vi "Mode Scan Engine.vi"() -> ()   [LabVIEW 2016]
uses:
  <vilib>/vision/Image Controls.llb/IMAQ Image.ctl
  Hardware Configuration/Hardware Configuration Controls/Standard Action.ctl
  Device Library/Cameras/Hamamatsu/Orca Flash/Orca Flash Controls/Orca Flash Actions.ctl
  Hardware Configuration/Hardware Configuration Controls/Device Type.ctl
  Hardware Configuration/Hardware Configuration Controls/Device Function.ctl
  Controls/Standard_Counter_Action.ctl
  Display Module/Display Module Custom Controls/ROI Descriptor.ctl
  Device Library/Cameras/Camera Controls/Camera IMAQ Key Info.ctl
  <vilib>/Analysis/baseanly.llb/Mean (DBL).vi
  <vilib>/Analysis/NI_AALBase.lvlib
  <vilib>/Analysis/NI_AALPro.lvlib
  <vilib>/Analysis/6fits.llb/Curve Fitting Criteria.ctl
  <vilib>/gmath/NI_Gmath.lvlib
  Device Library/Cameras/Photometrics/Prime BSI/Prime BSI Controls/Prime Actions.ctl
panel:
  in  "Accums":i32=1
  in  "Initial Guess":T1={"Amp"=7.0, "Center"=7.0, "Sigma"=7.0, "Offset"=7.0}
  in  "Manual Initial Guess":bool
  in  "Upper Limit":dbl=7.0
  in  "Lower Limit":dbl=7.0
  out "Metric":cluster{dbl[], dbl[]}[](graph)
  out "Image":u16[][](graph)
  in  "Step Size (nm)":u16=7
  in  "Number of Steps":u16=7
  in  "Get Image":bool
  in  "Scan Next Mode":bool
  in  "Metric":u16(ring) items=["Max Intensity", "No Zero Mean", "Threshold Mean"]
  in  "Fit Type":u16(ring) items=["Guassian", "Quadratic"]
  in  "Mode":i32(ring) items=["1", "2", "3", "4", "5", "6", "7", "8", "9", "10", "11", "12", "13", "14", "15", "16", "17", "18", "19", "20", "21", "22", "23", "24", "25", "26", "27", "28", "29", "30", "31", "32", "33", "34", "35", "36", "37", "38", "39", "40", "41", "42", "43", "44", "45", "46", "47", "48", "49", "50", "51", "52", "53", "54", "55", "56", "57", "58", "59", "60", "61", "62", "63", "64", "65", "66", "67", "68", "69", "70", "71", "72", "73", "74", "75", "76", "77", "78", "79", "80", "81", "82", "83", "84", "85", "86", "87", "88", "89", "90", "91", "92", "93", "94", "95", "96", "97", "98", "99", "100", "101", "102", "103", "104", "105", "106", "107", "108", "109", "110", "111", "112", "113", "114", "115", "116", "117", "118", "119", "120", "121", "122", "123", "124", "125", "126", "127", "128", "129", "130", "131", "132", "133", "134", "135", "136", "137", "138", "139", "140"]
  in  "Apply":bool
  in  "Fit Data":bool
  in  "Scan Mode":bool
  in  "Exit":bool
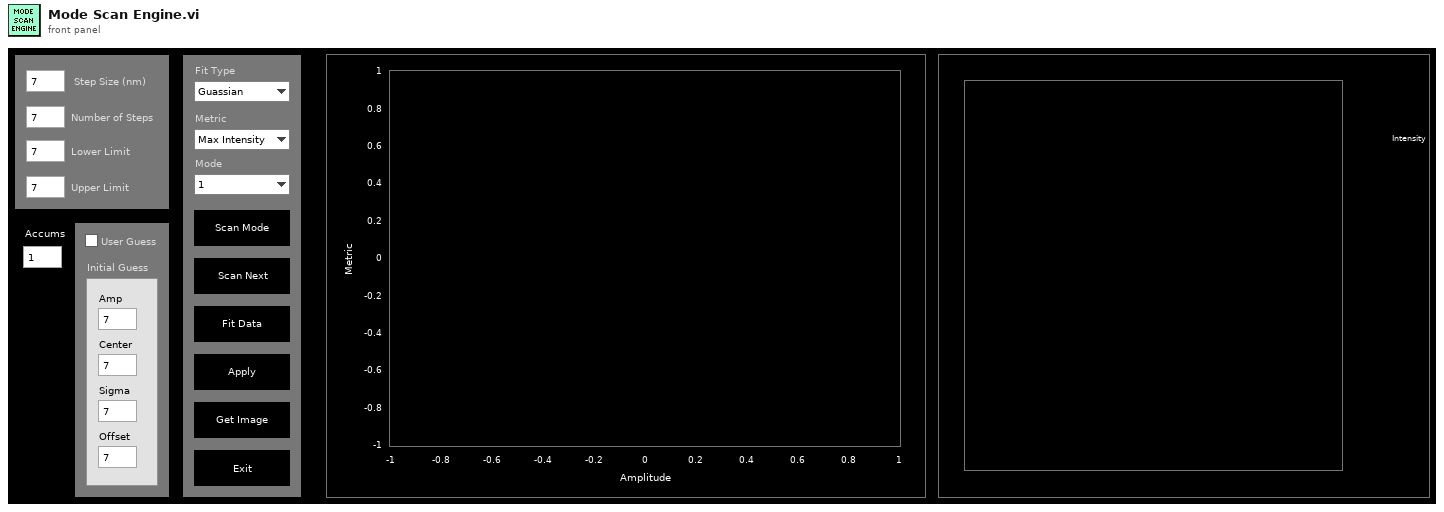
[diagram p1: front panel]
types:
  T1 = cluster{"Amp":dbl, "Center":dbl, "Sigma":dbl, "Offset":dbl}
  T2 = typedef "IMAQ Image.ctl" = refnum<image>
  T3 = typedef "Device Function.ctl" = enum16{"Primary", "Secondary", "Overview", "Wide Field Drift Correction", "642 nm Excitation", "560 nm Excitation", "546 nm Excitation", "488 nm Excitation", "405 nm Excitation", "Objective Drift Correction", "Objective XY", "Objective Z", "Sample XY", "Sample Coarse Z", "Sample Z", "4Pi Lower", "4Pi Upper", "Adj Cavity", "Line Scanning"}
  T4 = typedef "Device Type.ctl" = enum16{"AOTF", "Camera", "Deformable Mirror", "Laser", "Shutter", "Stage", "Waveform"}
  T5 = typedef "Orca Flash Actions.ctl" = enum16{"IDLE", "PREVIEW", "RECORD", "Record Settings", "SETPARAM", "GETPARAM", "SETROI", "GETROI", "PROGRESSIVE MODE", "AREA MODE", "STATUS", "QUIT"}
  T6 = typedef "Prime Actions.ctl" = enum16{"Error Check", "Initialize", "Preview", "Record", "Abort", "Record Settings", "Set Parameter", "Get Parameter", "Set ROI", "Get ROI", "Status", "Set Trigger", "Quit"}
  T7 = typedef "Standard Action.ctl" = enum16{"Read", "Write"}
  T8 = typedef "Standard_Counter_Action.ctl" = enum16{"Initialize", "Update Count", "Get Count"}
  T9 = typedef "ROI Descriptor.ctl" = cluster{"Global Rectangle":i32[], "Contours":cluster{"Contour Type":u32, "ROI Type":u32, "Points":i32[]}[]}
  T10 = typedef "Camera IMAQ Key Info.ctl" = cluster{"Frame":u32, "Sensor Height":i32, "Sensor Width":i32, "ROI Height":i32, "ROI Width":i32, "ROI Enable?":bool, "Bit per Pixel":u8}
  T11 = cluster{"amp min":dbl, "amp max":dbl, "center min":dbl, "center max":dbl, "deviation min":dbl, "deviation max":dbl, "offset min":dbl, "offset max":dbl}
  T12 = enum16{"Linear", "Polynomial", "Exponential", "Power"}
  T13 = typedef "MirrorModes.ctl" = cluster{"Mode":string, "Amplitude":dbl}[]
  T14 = cluster{"Amplitude Out":dbl[], "Metric Out":dbl[]}
  T15 = cluster{"Amp":dbl, "Numeric":dbl, "Sigma":dbl, "Offset":dbl}
  T16 = typedef "NI_AALPro.lvlib/Curve Fitting Criteria.ctl" = u16
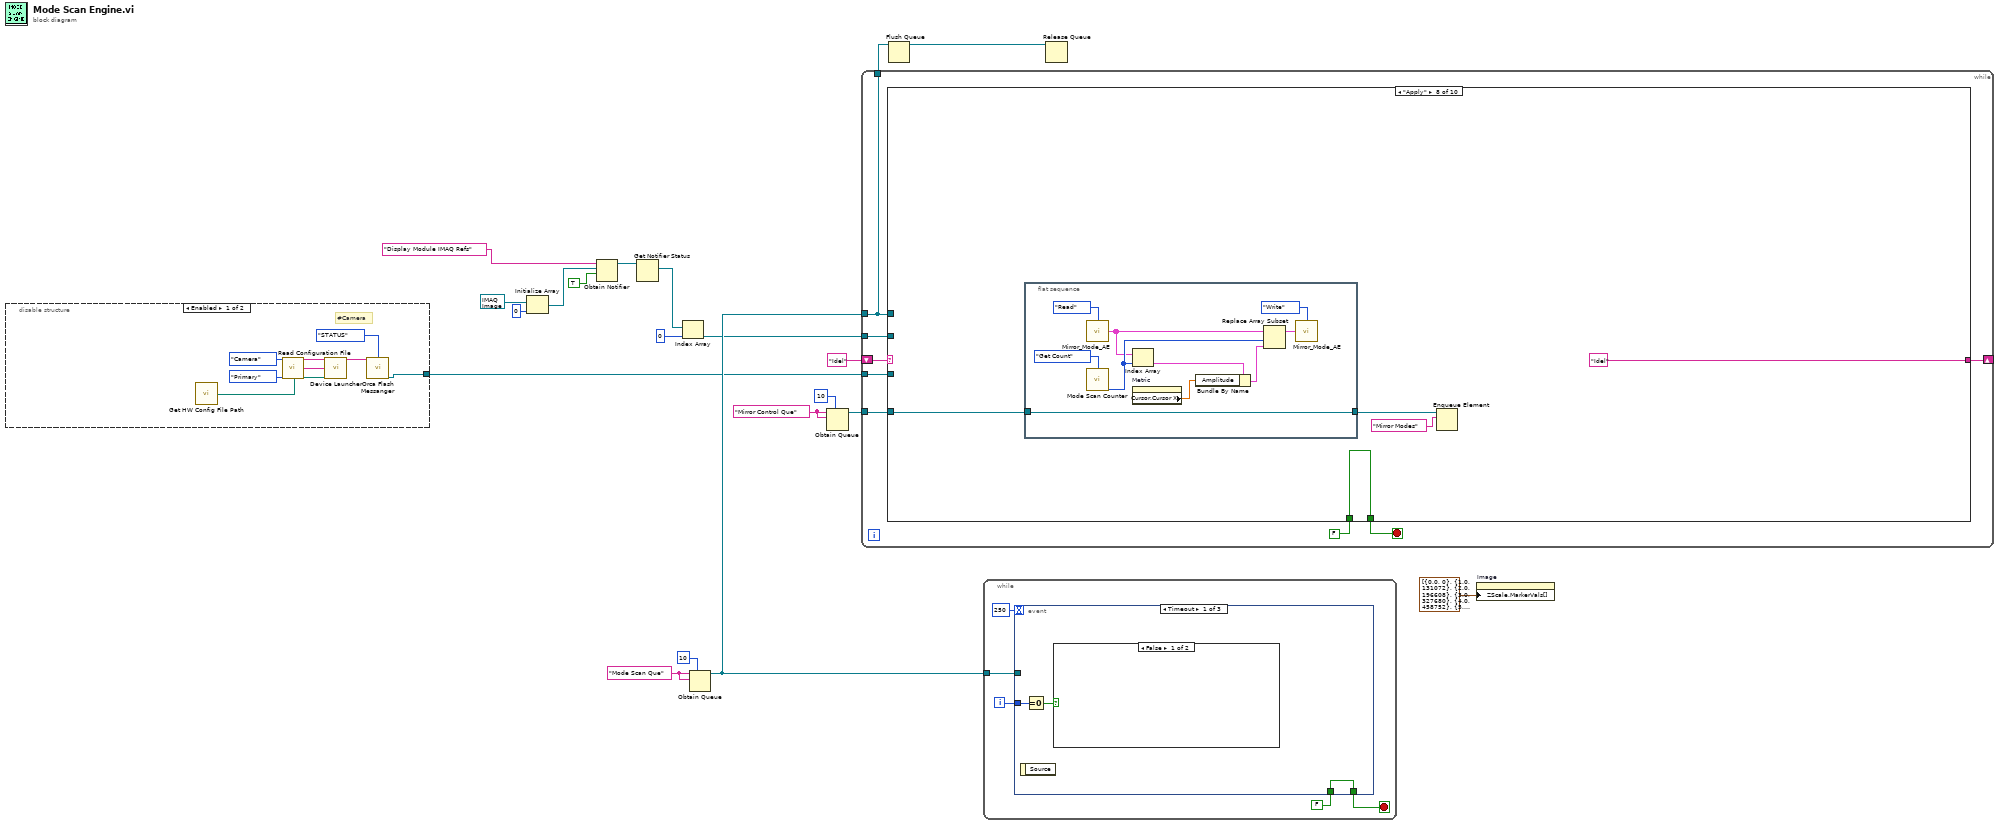
[diagram p0: block diagram]
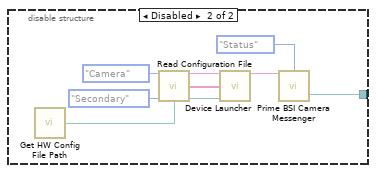
[diagram p2: hidden frame]
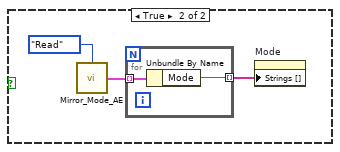
[diagram p3: hidden frame]
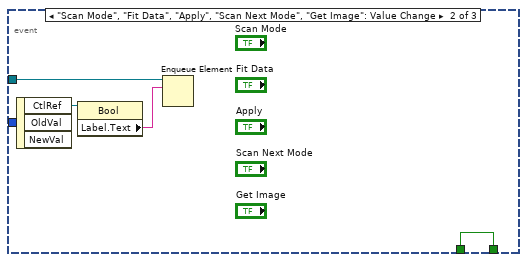
[diagram p4: hidden frame]
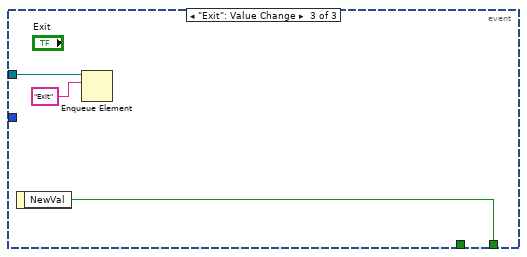
[diagram p5: hidden frame]
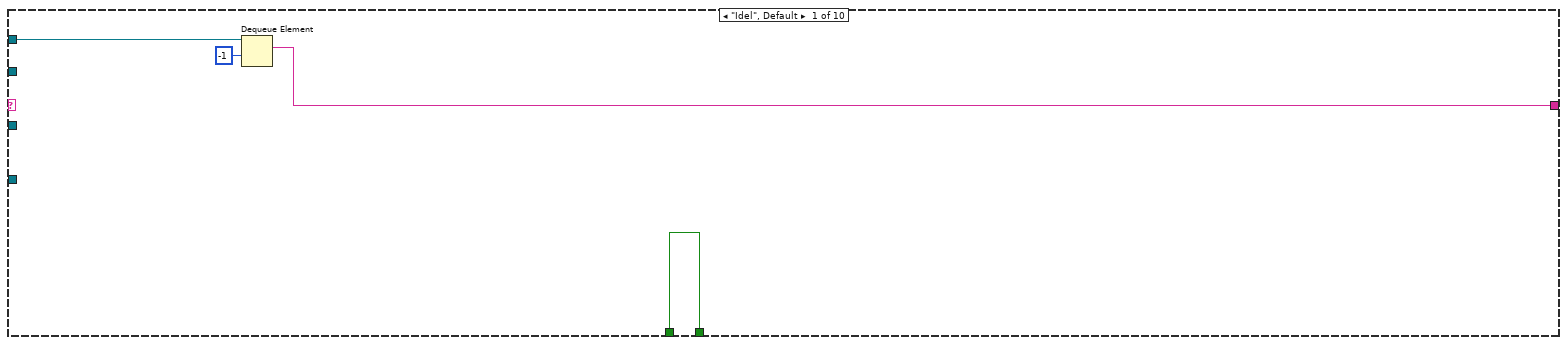
[diagram p6: hidden frame]
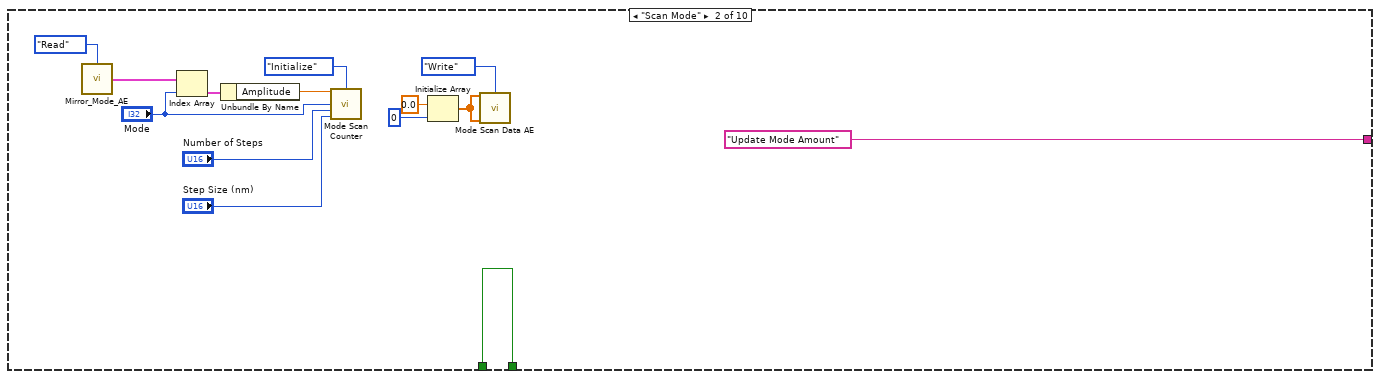
[diagram p7: hidden frame]
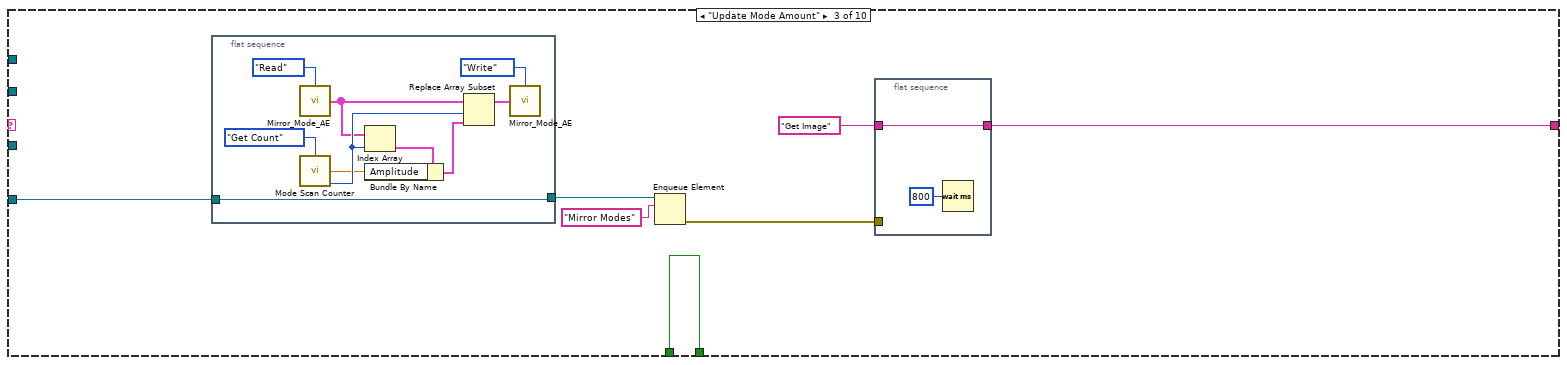
[diagram p8: hidden frame]
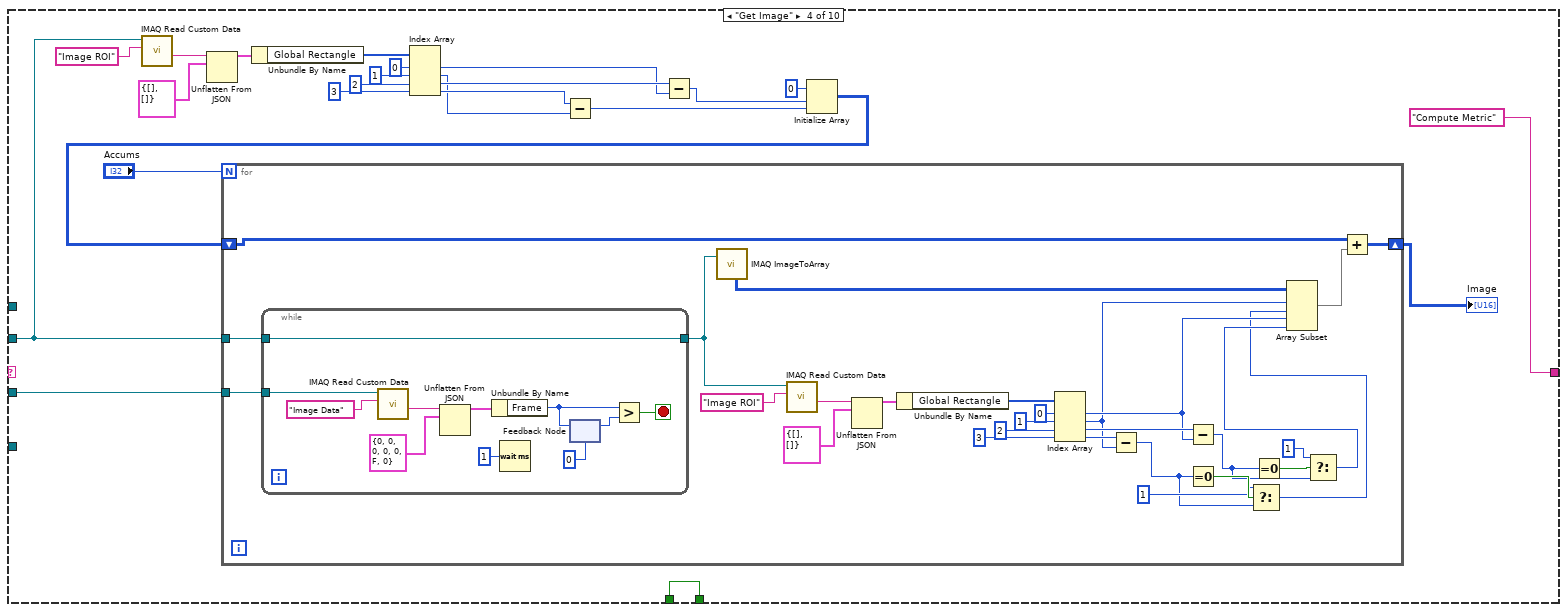
[diagram p9: hidden frame]
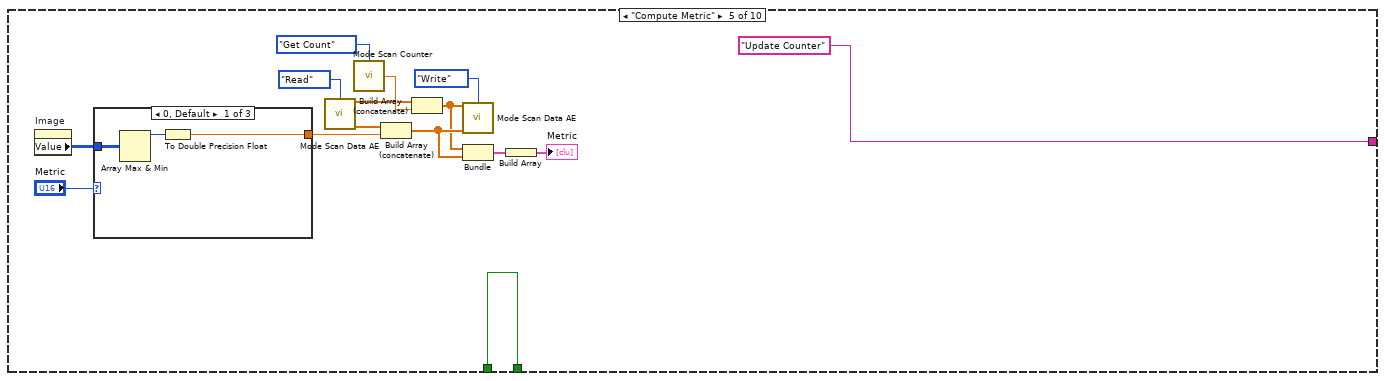
[diagram p10: hidden frame]
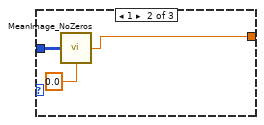
[diagram p11: hidden frame]
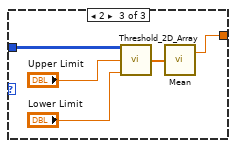
[diagram p12: hidden frame]
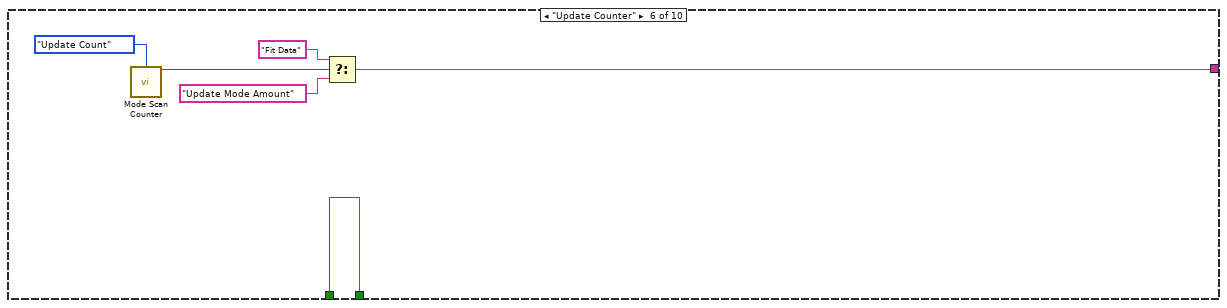
[diagram p13: hidden frame]
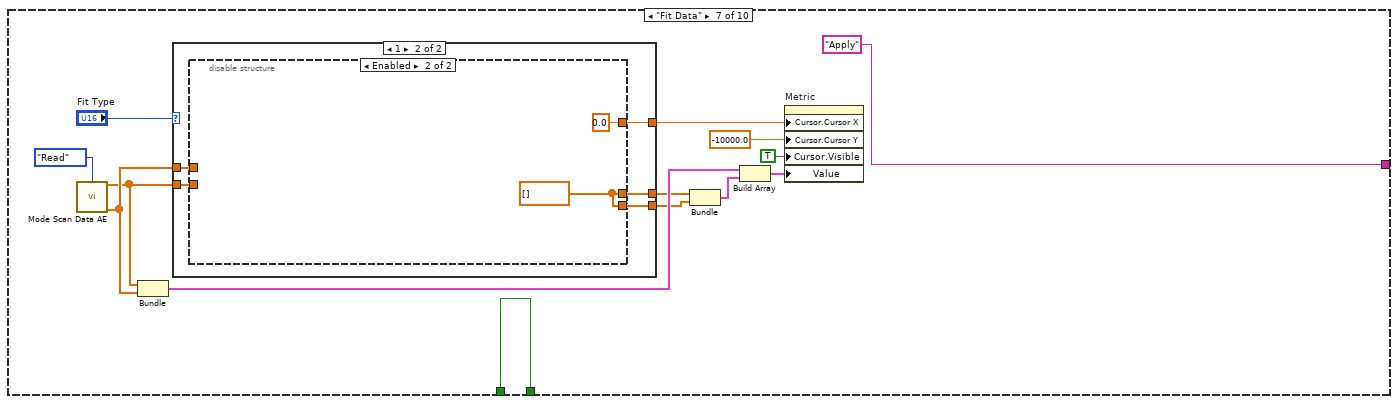
[diagram p14: hidden frame]
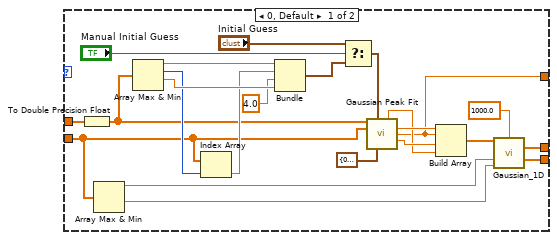
[diagram p15: hidden frame]
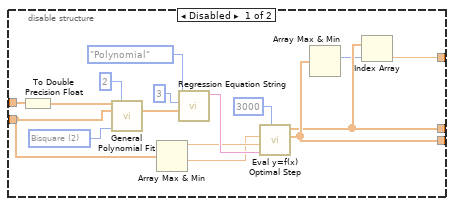
[diagram p16: hidden frame]
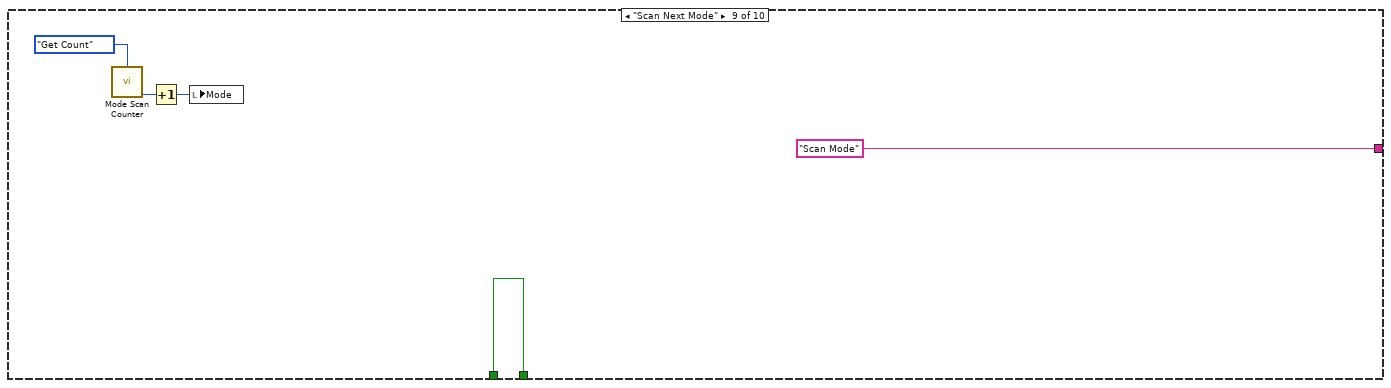
[diagram p17: hidden frame]
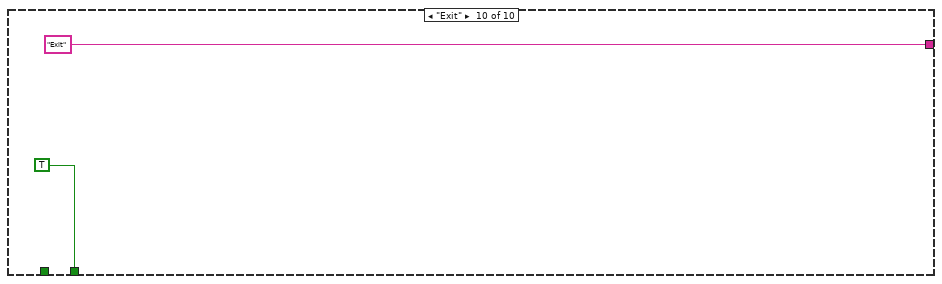
[diagram p18: hidden frame]
diagram:
  w14 = "Mirror Control Que" ("name (unnamed)")
  w19 = "Mode Scan Que" ("name (unnamed)")
  n1 = disable-structure shown="Enabled" {
    disable-tunnel: [w29 w31] -> w2
    frame Enabled {
      # "#Camera"
      n2 = call "Get HW Config File Path.vi"() -> ("File Path"=w22:path)  [unwired: 14 in, 1 out]
      n3 = call "Read Configuration File.vi"("Device Type"=Device_Type."Camera", "Device Function"=Device_Function."Primary", "Config File Path"=w22) -> ("Unique Notifier Name"=w23:string, "Device Ports/IDs/Channels"=w25:string[], "Device Engine Path"=w24:path)  [unwired: 9 in, 1 out]
      n4 = call "Device Launcher.vi"("Notifier Name"=w23, "Device Ports/IDs/Channels"=w25, "Device Engine Path"=w24) -> ("Notifier Name"=w21:string)  [unwired: 11 in, 1 out]
      n5 = call "Orca Flash Messanger.vi"("Notifier Name"=w21, "Camera Actions"=Orca_Flash_Actions."STATUS") -> ("Image Ref"=w29:T2)  [unwired: 9 in, 4 out]
    }
    frame Disabled {
      n6 = call "Get HW Config File Path.vi"() -> ("File Path"=w33:path)  [unwired: 14 in, 1 out]
      n7 = call "Read Configuration File.vi"("Device Type"=Device_Type."Camera", "Device Function"=Device_Function."Secondary", "Config File Path"=w33) -> ("Unique Notifier Name"=w34:string, "Device Ports/IDs/Channels"=w36:string[], "Device Engine Path"=w35:path)  [unwired: 9 in, 1 out]
      n8 = call "Device Launcher.vi"("Notifier Name"=w34, "Device Ports/IDs/Channels"=w36, "Device Engine Path"=w35) -> ("Notifier Name"=w32:string)  [unwired: 11 in, 1 out]
      n9 = call "Prime BSI Camera Messenger.vi"("Notifier Name"=w32, "Prime Actions"=Prime_Actions."Status") -> ("Image Ref"=w31:T2)  [unwired: 8 in, 5 out]
    }
  }
  n10 = Initialize Array(T2 refnum ("New Image"), 0 ("dimension size")) -> (w6:T2[])
  n11 = Obtain Notifier(name (unnamed)="Display Module IMAQ Refs", notification data type=w6, create if not found? (T)=TRUE) -> (notifier out=w5:refnum<notifier>)  [unwired: 1 in, 2 out]
  n12 = Get Notifier Status(notifier=w5) -> (current notification=w4:T2[])  [unwired: 1 in, 4 out]
  n13 = Index Array(array=w4, index=0) -> (element=w1:T2)
  n14 = Obtain Queue(max queue size (-1, unlimited)=10, name (unnamed)=w19, element data type=w19) -> (queue out=w17:refnum<queue>)  [unwired: 2 in, 2 out]
  n15 = Obtain Queue(max queue size (-1, unlimited)=10, name (unnamed)=w14, element data type=w14) -> (queue out=w12:refnum<queue>)  [unwired: 2 in, 2 out]
  n16 = while {
    shift-right: [w43] -> _
    shift-left: "Idel" -> [w46]
    tunnel: w17 -> [w42]
    tunnel: [w42] -> w16
    tunnel: w12 -> [w41]
    tunnel: w2 -> [w40]
    tunnel: w1 -> [w39]
    stop <- w45 stop-if-true
    n17 = case shown="\"Apply\"" w46 {
      tunnel: [w50 w64 w71 w106 w159 w177 w191 w242 w257 TRUE] -> w45
      tunnel: FALSE -> [w50 w64 w71 w106 w159 w177 w191 w242 w257 _]
      tunnel: w42 -> [w48 _ _ _ _ _ _ _ _ _]
      tunnel: [w47 "Update Mode Amount" ("name (unnamed)") w66 "Compute Metric" ("name (unnamed)") "Update Counter" ("name (unnamed)") w174 "Apply" ("name (unnamed)") "Idel" ("name (unnamed)") "Scan Mode" ("name (unnamed)") "Exit" ("name (unnamed)")] -> w43
      tunnel: w41 -> [_ _ w70 _ _ _ _ w240 _ _]
      tunnel: w40 -> [_ _ _ w104 _ _ _ _ _ _]
      tunnel: w39 -> [_ _ _ w93 _ _ _ _ _ _]
      frame "Idel", Default {
        n18 = Dequeue Element(queue=w48, timeout in ms (-1)=-1) -> (element=w47:string)  [unwired: 1 in, 3 out]
      }
      frame "Scan Mode" {
        n19 = call "Mirror_Mode_AE.vi"("Action"=Standard_Action."Read") -> ("Mirror Modes Out"=w59:T13)  [unwired: 14 in]
        n20 = Index Array(array=w59, index="Mode") -> (element=w60:cluster{"Mode":string, "Amplitude":dbl})
        n21 = Unbundle By Name(w60) -> ("Amplitude"=w61:dbl)
        n22 = call "Mode Scan Counter.vi"("Center Value"=w61, "Action"=Standard_Counter_Action."Initialize", "Mode"="Mode", "Number of Steps"="Number of Steps", "Step Size"="Step Size (nm)") -> ()  [unwired: 8 in, 3 out]
        n23 = Initialize Array(0.0 ("element"), 0 ("dimension size")) -> (w51:dbl[])
        n24 = call "Mode Scan Data AE.vi"("Amplitude"=w51, "Action"=Standard_Action."Write", "Metric"=w51) -> ()  [unwired: 11 in, 2 out]
      }
      frame "Update Mode Amount" {
        n25 = flat-sequence {
          tunnel: w70 -> [w74]
          tunnel: [w74] -> w68
          frame #0 {
            n26 = call "Mirror_Mode_AE.vi"("Action"=Standard_Action."Read") -> ("Mirror Modes Out"=w77:T13)  [unwired: 14 in]
            n27 = call "Mode Scan Counter.vi"("Action"=Standard_Counter_Action."Get Count") -> ("Output"=w81:dbl, "Current Mode"=w82:i32)  [unwired: 12 in, 1 out]
            n28 = Index Array(array=w77, index=w82) -> (element=w80:cluster{"Mode":string, "Amplitude":dbl})
            n29 = Bundle By Name(cluster=w80, "Amplitude"=w81) -> (w83:cluster{"Mode":string, "Amplitude":dbl})
            n30 = Replace Array Subset(array=w77, new element=w83, index=w82) -> (w79:T13)
            n31 = call "Mirror_Mode_AE.vi"("Action"=Standard_Action."Write", "Mirror Modes In"=w79) -> ()  [unwired: 13 in, 1 out]
          }
        }
        n32 = Enqueue Element(queue=w68, element="Mirror Modes" ("name (unnamed)")) -> (error out=w65:errorcluster)  [unwired: 2 in, 2 out]
        n33 = flat-sequence {
          tunnel: "Get Image" ("name (unnamed)") -> [w72]
          tunnel: [w72] -> w66
          tunnel: w65 -> [_]
          frame #0 {
            n34 = Wait (ms)(milliseconds to wait=u32 800) -> ()  [unwired: 1 out]
          }
        }
      }
      frame "Get Image" {
        n35 = call "IMAQ Read Custom Data"("Key"="Image ROI", "Image"=w93) -> ("Custom Data Out"=w95:string)  [unwired: 7 in, 2 out]
        n36 = Unflatten From JSON(JSON string=w95, type and defaults=T9 {"Global Rectangle"=[], "Contours"=[]} ("Image ROI Descriptor")) -> (value=w97:T9)  [unwired: 5 in, 1 out]
        n37 = Unbundle By Name(w97) -> ("Global Rectangle"=w98:i32[])
        n38 = Index Array(array=w98, index #1=0 ("index"), index #2=1 ("index"), index #3=2 ("index"), index #4=3 ("index")) -> (element #1=w91:i32, element #2=w84:i32, element #3=w92:i32, element #4=w85:i32)
        n39 = Subtract(x=w85, y=w84) -> (x-y=w89:i32)
        n40 = Subtract(x=w92, y=w91) -> (x-y=w90:i32)
        n41 = Initialize Array(u16 0 ("element"), w90, w89) -> (w87:u16[][])
        n42 = for {
          N: "Accums" -> [_]
          tunnel: w104 -> [w134]
          tunnel: w93 -> [w133]
          shift-right: [w108] -> w86
          shift-left: w87 -> [w107]
          n43 = while {
            tunnel: w134 -> [w138]
            tunnel: w133 -> [w135]
            tunnel: [w135] -> w129
            stop <- w137 stop-if-true
            n44 = call "IMAQ Read Custom Data"("Key"="Image Data", "Image"=w138) -> ("Custom Data Out"=w144:string)  [unwired: 7 in, 2 out]
            n45 = Unflatten From JSON(JSON string=w144, type and defaults=T10 {"Frame"=0, "Sensor Height"=0, "Sensor Width"=0, "ROI Height"=0, "ROI Width"=0, "ROI Enable?"=FALSE, "Bit per Pixel"=0} ("Camera IMAQ Key Info")) -> (value=w142:T10)  [unwired: 5 in, 1 out]
            n46 = Unbundle By Name(w142) -> ("Frame"=w141:u32)
            n47 = Wait (ms)(milliseconds to wait=u32 1) -> ()  [unwired: 1 out]
            n48 = feedback #1(u32 0 ("Frame")) -> (w140:u32)
            n49 = feedback-in #1(w141) -> ()
            n50 = Greater?(x=w141, y=w140) -> (0:w137:bool)
          }
          n51 = call "IMAQ ImageToArray"("Image"=w129) -> ("Image Pixels (U16)"=w122:u16[][])  [unwired: 3 in, 4 out]
          n52 = call "IMAQ Read Custom Data"("Key"="Image ROI", "Image"=w129) -> ("Custom Data Out"=w131:string)  [unwired: 7 in, 2 out]
          n53 = Unflatten From JSON(JSON string=w131, type and defaults=T9 {"Global Rectangle"=[], "Contours"=[]} ("Image ROI Descriptor")) -> (value=w128:T9)  [unwired: 5 in, 1 out]
          n54 = Unbundle By Name(w128) -> ("Global Rectangle"=w127:i32[])
          n55 = Index Array(array=w127, index #1=0 ("index"), index #2=1 ("index"), index #3=2 ("index"), index #4=3 ("index")) -> (element #1=w119:i32, element #2=w118:i32, element #3=w121:i32, element #4=w120:i32)
          n56 = Subtract(x=w120, y=w118) -> (x-y=w113:i32)
          n57 = Subtract(x=w121, y=w119) -> (x-y=w112:i32)
          n58 = Equal To 0?(x=w113) -> (x = 0?=w117:bool)
          n59 = Select(t=1 ("index"), s=w117, f=w113) -> (s? t:f=w110:i32)
          n60 = Equal To 0?(x=w112) -> (x = 0?=w116:bool)
          n61 = Select(t=1 ("index"), s=w116, f=w112) -> (s? t:f=w111:i32)
          n62 = Array Subset(array=w122, index (row)=w118, length (row)=w110, index (col)=w119, length (col)=w111) -> (w109:u16[][])
          n63 = Add(x=w107, y=w109) -> (x+y=w108:u16[][])
        }
        "Image" <- w86
      }
      frame "Compute Metric" {
        n64 = property on="Image" class="IntGraph (strict)"() -> ("Value"=w146:u16[][])  [unwired: 2 in, 2 out]
        n65 = case shown="0, Default" "Metric" {
          tunnel: w146 -> [w163 w166 w171]
          tunnel: [w161 w165 w169] -> w153
          frame 0, Default {
            n66 = Array Max & Min(array=w163) -> (max value=w162:u16)  [unwired: 3 out]
            n67 = To Double Precision Float(number=w162) -> (double precision float=w161:dbl)
          }
          frame 1 {
            n68 = call "MeanImage_NoZeros.vi"("Image IN"=w166, "STDev Factor"=0.0) -> ("No Zero Mean"=w165:dbl)  [unwired: 13 in]
          }
          frame 2 {
            n69 = call "Threshold_2D_Array.vi"("2D Array IN"=w171, "Upper Limit"="Upper Limit", "Lower Limit"="Lower Limit") -> ("Threshold Array Out"=w170:dbl[])  [unwired: 12 in]
            n70 = call-poly <vilib>:"Mean.vi"("X"=w170) -> ("mean"=w169:dbl)  [unwired: 1 out]
          }
        }
        n71 = call "Mode Scan Data AE.vi"("Action"=Standard_Action."Read") -> ("Amplitude Out"=w150:dbl[], "Metric Out"=w151:dbl[])  [unwired: 13 in]
        n72 = call "Mode Scan Counter.vi"("Action"=Standard_Counter_Action."Get Count") -> ("Output"=w152:dbl)  [unwired: 12 in, 2 out]
        n73 = Build Array (concatenate)(w151, w153) -> (w156:dbl[])
        n74 = Build Array (concatenate)(w150, w152) -> (w155:dbl[])
        n75 = call "Mode Scan Data AE.vi"("Amplitude"=w155, "Action"=Standard_Action."Write", "Metric"=w156) -> ()  [unwired: 11 in, 2 out]
        n76 = Bundle(w155, w156) -> (w157:cluster{dbl[], dbl[]})  [unwired: 1 in]
        n77 = Build Array(w157) -> (→"Metric":cluster{dbl[], dbl[]}[])
      }
      frame "Update Counter" {
        n78 = call "Mode Scan Counter.vi"("Action"=Standard_Counter_Action."Update Count") -> ("Scan Done?"=w172:bool)  [unwired: 12 in, 2 out]
        n79 = Select(t="Fit Data", s=w172, f="Update Mode Amount") -> (s? t:f=w174:string)
      }
      frame "Fit Data" {
        n80 = call "Mode Scan Data AE.vi"("Action"=Standard_Action."Read") -> ("Amplitude Out"=w186:dbl[], "Metric Out"=w187:dbl[])  [unwired: 13 in]
        n81 = Bundle("Amplitude Out"=w186, "Metric Out"=w187) -> (w185:T14)  [unwired: 1 in]
        n82 = case shown="1" "Fit Type" {
          tunnel: w186 -> [w207 w219]
          tunnel: w187 -> [w214 w218]
          tunnel: [w195 w215] -> w180
          tunnel: [w194 w216] -> w183
          tunnel: [w193 w217] -> w182
          frame 0, Default {
            n83 = To Double Precision Float(number=w214) -> (double precision float=w208:dbl[])
            n84 = Array Max & Min(array=w207) -> (max value=w196:dbl, min value=w197:dbl)  [unwired: 2 out]
            n85 = Array Max & Min(array=w208) -> (max value=w213:dbl, max index (indices)=w210:i32, min value=w212:dbl)  [unwired: 1 out]
            n86 = Index Array(array=w207, index=w210) -> (element=w209:dbl)
            n87 = Bundle(w213, "Numeric"=w209, 4.0, w212) -> (w206:cluster{dbl, "Numeric":dbl, dbl, dbl})  [unwired: 1 in]
            n88 = Select(t="Initial Guess", s="Manual Initial Guess", f=w206) -> (s? t:f=w205:T15)
            n89 = call <vilib>:"Gaussian Peak Fit.vi"("Y"=w208, "initial guess"=w205, "X"=w207, "parameter bounds"=T11 {"amp min"=0.0, "amp max"=100000.0, "center min"=-100.0, "center max"=100.0, "deviation min"=0.0, "deviation max"=1000.0, "offset min"=0.0, "offset max"=1000.0}) -> ("offset"=w200:dbl, "amplitude"=w202:dbl, "center"=w195:dbl, "standard deviation"=w201:dbl)  [unwired: 5 in, 3 out]
            n90 = Build Array(w202, w195, w201, w200) -> (w199:dbl[])
            n91 = call "Gaussian_1D.vi"("Parameters In"=w199, "Number of Points"=1000.0, "Max X Value"=w196, "Min X Value"=w197) -> ("X Values"=w194:dbl[], "Y Values"=w193:dbl[])  [unwired: 10 in]
          }
          frame 1 {
            n92 = disable-structure shown="Enabled" {
              disable-tunnel: w219 -> [w225 _]
              disable-tunnel: w218 -> [w224 _]
              disable-tunnel: [w223 w236] -> w217
              disable-tunnel: [w222 w236] -> w216
              disable-tunnel: [w221 0.0] -> w215
              frame Disabled {
                w234 = T16 2 items=["Least Square", "Least Absolute Residual", "Bisquare"] ("method")
                n93 = To Double Precision Float(number=w224) -> (double precision float=w235:dbl[])
                n94 = call <vilib>:"General Polynomial Fit.vi"("Y"=w235, "polynomial order"=2, "X"=w225, "method"=w234) -> ("Polynomial Coefficients"=w231:dbl[])  [unwired: 8 in, 3 out]
                n95 = Array Max & Min(array=w225) -> (max value=w227:dbl, min value=w226:dbl)  [unwired: 2 out]
                n96 = call "Regression Equation String.vi"("coefficients"=w231, "precision"=3, "fit type"=T12."Polynomial") -> ("Formula"=w229:string)  [unwired: 8 in]
                n97 = call <vilib>:"Eval y=f(x) Optimal Step.vi"("number of points"=u32 3000, "formula"=w229, "end"=w227, "start"=w226) -> ("Y Values"=w223:dbl[], "X Values"=w222:dbl[])  [unwired: 1 in, 2 out]
                n98 = Array Max & Min(array=w223) -> (max index (indices)=w220:i32)  [unwired: 3 out]
                n99 = Index Array(array=w222, index=w220) -> (element=w221:dbl)
              }
              frame Enabled {
                w236 = dbl[] [] ("X Values")
              }
            }
          }
        }
        n100 = Bundle("X Values"=w183, "X Values"=w182) -> (w181:cluster{"X Values":dbl[], "X Values":dbl[]})  [unwired: 1 in]
        n101 = Build Array(w185, w181) -> (w184:cluster{"X Values":dbl[], "X Values":dbl[]}[])
        n102 = property on="Metric" class="XYGraph (strict)"("Cursor.Cursor X"=w180, "Cursor.Cursor Y"=-10000.0 ("Cursor.Cursor Position:Cursor X"), "Cursor.Visible"=TRUE, "Value"=w184) -> ()  [unwired: 2 in, 2 out]
      }
      frame "Apply" {
        n103 = flat-sequence {
          tunnel: [w244] -> w238
          tunnel: w240 -> [w244]
          frame #0 {
            n104 = call "Mirror_Mode_AE.vi"("Action"=Standard_Action."Read") -> ("Mirror Modes Out"=w247:T13)  [unwired: 14 in]
            n105 = call "Mode Scan Counter.vi"("Action"=Standard_Counter_Action."Get Count") -> ("Current Mode"=w251:i32)  [unwired: 12 in, 2 out]
            n106 = Index Array(array=w247, index=w251) -> (element=w250:cluster{"Mode":string, "Amplitude":dbl})
            n107 = property on="Metric" class="XYGraph (strict)"() -> ("Cursor.Cursor X"=w243:dbl)  [unwired: 2 in, 2 out]
            n108 = Bundle By Name(cluster=w250, "Amplitude"=w243) -> (w252:cluster{"Mode":string, "Amplitude":dbl})
            n109 = Replace Array Subset(array=w247, new element=w252, index=w251) -> (w249:T13)
            n110 = call "Mirror_Mode_AE.vi"("Action"=Standard_Action."Write", "Mirror Modes In"=w249) -> ()  [unwired: 13 in, 1 out]
          }
        }
        n111 = Enqueue Element(queue=w238, element="Mirror Modes" ("name (unnamed)")) -> ()  [unwired: 2 in, 3 out]
      }
      frame "Scan Next Mode" {
        n112 = call "Mode Scan Counter.vi"("Action"=Standard_Counter_Action."Get Count") -> ("Current Mode"=w254:i32)  [unwired: 12 in, 2 out]
        n113 = Increment(x=w254) -> (x+1=w255:i32)
        n114 = local write "Mode"(w255) -> ()
      }
      frame "Exit" {
      }
    }
  }
  n115 = Flush Queue(queue=w16) -> (queue out=w15:refnum<queue>)  [unwired: 1 in, 2 out]
  n116 = while {
    tunnel: w17 -> [w264]
    i -> [w261]
    stop <- w263 stop-if-true
    n117 = event shown="[0] Timeout" {
      selector: _ -> [_ _ _]
      dyn-events: _ -> [_ _ _]
      timeout: 250 -> [_ _ _]
      tunnel: w264 -> [_ w275 w279]
      tunnel: [w267 w273 w277] -> w263
      tunnel: FALSE -> [w267 w273 _]
      tunnel: w261 -> [w266 _ _]
      event Timeout {
        n118 = event-data() -> ()  [unwired: 1 in, 1 out]
        n119 = Equal To 0?(x=w266) -> (x = 0?=w265:bool)
        n120 = case shown="False" w265 {
          frame False {
          }
          frame True {
            n121 = call "Mirror_Mode_AE.vi"("Action"=Standard_Action."Read") -> ("Mirror Modes Out"=w269:T13)  [unwired: 14 in]
            n122 = for {
              tunnel: w269 -> [w272] mode=indexing
              tunnel: [w271] -> w270 mode=indexing
              n123 = Unbundle By Name(w272) -> ("Mode"=w271:string)
            }
            n124 = property on="Mode" class="Ring (strict)"("Strings []"=w270) -> ()  [unwired: 2 in, 2 out]
          }
        }
      }
      event "Scan Mode", "Fit Data", "Apply", "Scan Next Mode", "Get Image": Value Change {
        n125 = event-data() -> ("CtlRef"=w274:refnum<vi>)  [unwired: 1 in, 2 out]
        n126 = property class="Bool"(reference=w274) -> ("Label.Text"=w276:string)  [unwired: 1 in, 2 out]
        n127 = Enqueue Element(queue=w275, element=w276) -> ()  [unwired: 2 in, 3 out]
      }
      event "Exit": Value Change {
        n128 = event-data() -> ("NewVal"=w277:bool)  [unwired: 1 in]
        n129 = Enqueue Element(queue=w279, element="Exit") -> ()  [unwired: 2 in, 3 out]
      }
    }
  }
  n130 = Release Queue(queue=w15) -> ()  [unwired: 2 in, 3 out]
  n131 = property on="Image" class="IntGraph (strict)"("ZScale.MarkerVals[]"=cluster{dbl, u32}[] [{0.0, 0}, {1.0, 131072}, {2.0, 196608}, {3.0, 327680}, {4.0, 458752}, {5.0, 589824}, {6.0, 720896}, {7.0, 851971}, {8.0, 983043}, {9.0, 1114115}, {10.0, 1245187}, {11.0, 1376259}, {12.0, 1507331}, {13.0, 1638403}, {14.0, 1769475}, {15.0, 1769479}, {16.0, 2031623}, {17.0, 2162695}, {18.0, 2293767}, {19.0, 2424839}, {20.0, 2555911}, {21.0, 2686983}, {22.0, 2818055}, {23.0, 2949127}, {24.0, 3080203}, {25.0, 3211275}, {26.0, 3342347}, {27.0, 3473419}, {28.0, 3604491}, {29.0, 3735563}, {30.0, 3866635}, {31.0, 3867403}, {32.0, 4129547}, {33.0, 4260619}, {34.0, 4391691}, {35.0, 4522763}, {36.0, 4653839}, {37.0, 4784911}, {38.0, 4915983}, {39.0, 5178127}, {40.0, 5309199}, {41.0, 5440271}, {42.0, 5571343}, {43.0, 5702415}, {44.0, 5703439}, {45.0, 5965583}, {46.0, 6096655}, {47.0, 6227727}, {48.0, 6358799}, {49.0, 6489871}, {50.0, 6620943}, {51.0, 6752015}, {52.0, 6883087}, {53.0, 7015183}, {54.0, 7146255}, {55.0, 7277327}, {56.0, 7408399}, {57.0, 7539471}, {58.0, 7670543}, {59.0, 7801615}, {60.0, 8063759}, {61.0, 8194831}, {62.0, 8326927}, {63.0, 8457999}, {64.0, 8589075}, {65.0, 8720147}, {66.0, 8851219}, {67.0, 8982291}, {68.0, 9113363}, {69.0, 9114387}, {70.0, 9376531}, {71.0, 9507603}, {72.0, 9638675}, {73.0, 9769747}, {74.0, 9901843}, {75.0, 10032915}, {76.0, 10163987}, {77.0, 10229523}, {78.0, 10295059}, {79.0, 10427155}, {80.0, 10558227}, {81.0, 10689299}, {82.0, 10820371}, {83.0, 10886931}, {84.0, 10952467}, {85.0, 11083539}, {86.0, 11214611}, {87.0, 11215635}, {88.0, 11477779}, {89.0, 11543315}, {90.0, 11608851}, {91.0, 11740947}, {92.0, 11806483}, {93.0, 11872019}, {94.0, 12004115}, {95.0, 12135187}, {96.0, 12266259}, {97.0, 12267283}, {98.0, 12398355}, {99.0, 12529427}, {100.0, 12530451}, {101.0, 12595987}, {102.0, 12530451}, {103.0, 12793619}, {104.0, 12794131}, {105.0, 12794643}, {106.0, 13056787}, {107.0, 13057299}, {108.0, 13057811}, {109.0, 13188883}, {110.0, 13320979}, {111.0, 13386515}, {112.0, 13452563}, {113.0, 13584147}, {114.0, 13584659}, {115.0, 13585171}, {116.0, 13585683}, {117.0, 13717267}, {118.0, 13848339}, {119.0, 13849363}, {120.0, 13849875}, {121.0, 13850387}, {122.0, 13981459}, {123.0, 14113555}, {124.0, 14114067}, {125.0, 14114579}, {126.0, 14115091}, {127.0, 14246675}, {128.0, 14377747}, {129.0, 14378771}, {130.0, 14379283}, {131.0, 14379539}, {132.0, 14379795}, {133.0, 14380819}, {134.0, 14511891}, {135.0, 14643987}, {136.0, 14644503}, {137.0, 14645015}, {138.0, 14645527}, {139.0, 14646039}, {140.0, 14646551}, {141.0, 14778135}, {142.0, 14909207}, {143.0, 14910231}, {144.0, 14910747}, {145.0, 14911259}, {146.0, 14911771}, {147.0, 14912283}, {148.0, 14912797}, {149.0, 15044383}, {150.0, 15175455}, {151.0, 15175967}, {152.0, 15176479}, {153.0, 15176991}, {154.0, 15177507}, {155.0, 15178019}, {156.0, 15178531}, {157.0, 15310115}, {158.0, 15441701}, {159.0, 15441959}, {160.0, 15442215}, {161.0, 15442727}, {162.0, 15443243}, {163.0, 15443755}, {164.0, 15444269}, {165.0, 15444783}, {166.0, 15444783}, {167.0, 15576367}, {168.0, 15707953}, {169.0, 15708467}, {170.0, 15708979}, {171.0, 15708981}, {172.0, 15708983}, {173.0, 15710011}, {174.0, 15710523}, {175.0, 15711037}, {176.0, 15711039}, {177.0, 15711553}, {178.0, 15843139}, {179.0, 15974213}, {180.0, 15974215}, {181.0, 15974217}, {182.0, 15974219}, {183.0, 15975755}, {184.0, 15976271}, {185.0, 15976785}, {186.0, 15977299}, {187.0, 15977301}, {188.0, 15977815}, {189.0, 15978327}, {190.0, 15978331}, {191.0, 16109917}, {192.0, 16241503}, {193.0, 16241505}, {194.0, 16242019}, {195.0, 16242535}, {196.0, 16242537}, {197.0, 16242539}, {198.0, 16243563}, {199.0, 16243567}, {200.0, 16244081}, {201.0, 16244595}, {202.0, 16244599}, {203.0, 16244601}, {204.0, 16244603}, {205.0, 16245627}, {206.0, 16245631}, {207.0, 16245633}, {208.0, 16246147}, {209.0, 16246663}, {210.0, 16377735}, {211.0, 16508811}, {212.0, 16508815}, {213.0, 16509839}, {214.0, 16509843}, {215.0, 16509845}, {216.0, 16509847}, {217.0, 16510361}, {218.0, 16510875}, {219.0, 16510879}, {220.0, 16510881}, {221.0, 16510883}, {222.0, 16511399}, {223.0, 16511911}, {224.0, 16511915}, {225.0, 16511917}, {226.0, 16511919}, {227.0, 16511923}, {228.0, 16512437}, {229.0, 16512951}, {230.0, 16512955}, {231.0, 16512957}, {232.0, 16512959}, {233.0, 16512961}, {234.0, 16512963}, {235.0, 16512967}, {236.0, 16513481}, {237.0, 16513995}, {238.0, 16513999}, {239.0, 16514001}, {240.0, 16514003}, {241.0, 16514005}, {242.0, 16514007}, {243.0, 16514011}, {244.0, 16514013}, {245.0, 16514015}, {246.0, 16514019}, {247.0, 16514021}, {248.0, 16514023}, {249.0, 16514027}, {250.0, 16514029}, {251.0, 16514031}, {252.0, 16514035}, {253.0, 16514037}, {254.0, 16514039}, {255.0, 16514043}] ("Z Scale.Marker Values[]")) -> ()  [unwired: 2 in, 2 out]
